vi "Write String.vi"(8 "error in (no error)":errorcluster, 9 "String":string, 10 "VISA resource name in":refnum<visa-resource-name>, 11 "LCD-I2C in":refnum<class "LCD-I2C.lvclass">) -> (0 "error out":errorcluster, 2 "VISA resource name":refnum<visa-resource-name>, 3 "LCD-I2C out":refnum<class "LCD-I2C.lvclass">)   [LabVIEW 2020, in "CTI-Visa-DeviceLib.lvlib" / "LCD-I2C.lvclass"]
uses:
  LCD-I2C.lvclass
  LCD-I2C.lvclass/LCD-I2C.ctl
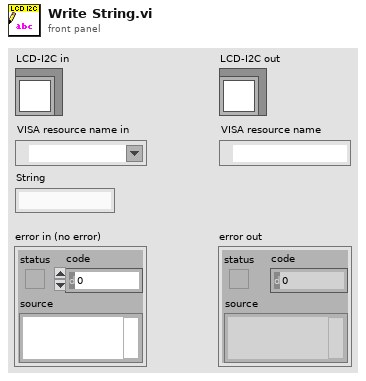
[diagram p1: front panel]
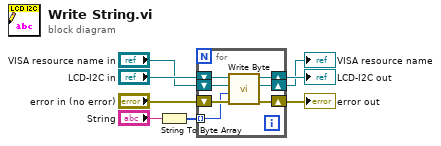
[diagram p0: block diagram]
diagram:
  n1 = String To Byte Array(string="String") -> (unsigned byte array=w1:u8[])
  n2 = for {
    shift-right: [w14] -> w6
    shift-left: "error in (no error)" -> [w15]
    shift-right: [w12] -> w4
    shift-left: "LCD-I2C in" -> [w13]
    shift-right: [w10] -> w2
    shift-left: "VISA resource name in" -> [w11]
    tunnel: w1 -> [w9] mode=indexing
    n3 = call "Write Byte.vi"("error in (no error)"=w15, "Value"=w9, "VISA resource name in"=w11, "LCD-I2C in"=w13) -> ("error out"=w14:errorcluster, "VISA resource name"=w10:refnum<visa-resource-name>, "LCD-I2C out"=w12:refnum<class "LCD-I2C.lvclass">)  [unwired: 5 in]
  }
  "error out" <- w6
  "LCD-I2C out" <- w4
  "VISA resource name" <- w2
